vi "Cimb Set Modes.vi"   [LabVIEW 2016]
uses:
  Climb Control Type.ctl
  Climb Globals.vi
types:
  T1 = typedef "Climb Control Type.ctl" = enum16{"No Op", "Up", "Down"}
  T2 = typedef "Climb Notifier.ctl" = cluster{"Up":bool, "Down":bool, "Climb Control List":T1}
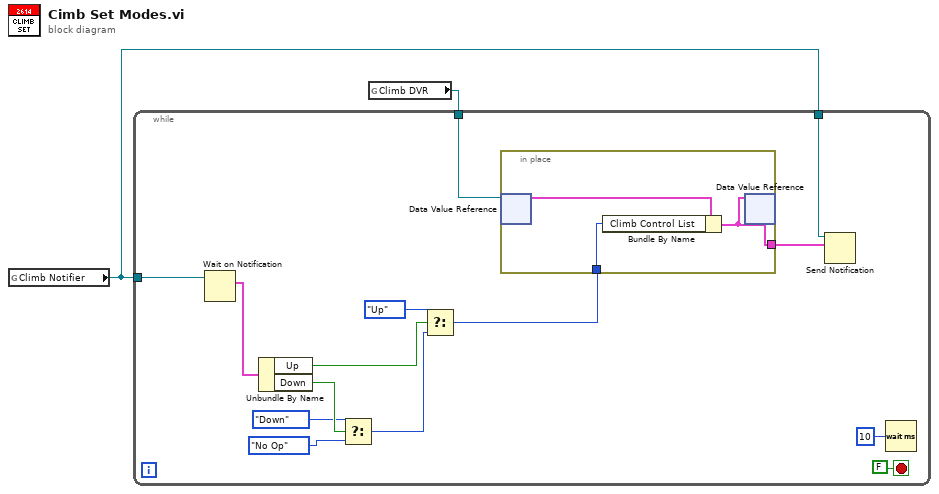
[diagram p0: block diagram]
diagram:
  n1 = global read "Climb Globals.vi" "Climb Notifier"() -> (w1:refnum<notifier>)
  n2 = global read "Climb Globals.vi" "Climb DVR"() -> (w2:refnum<data-value>)
  n3 = while {
    tunnel: w1 -> [w10]
    tunnel: w2 -> [w9]
    tunnel: w1 -> [w6]
    stop <- FALSE stop-if-true
    n4 = Wait on Notification(notifier=w10) -> (notification=w14:T2)  [unwired: 3 in, 3 out]
    n5 = Unbundle By Name(w14) -> ("Up"=w13:bool, "Down"=w12:bool)
    n6 = Select(t=Climb_Control_Type."Down" ("Climb Control List"), s=w12, f=Climb_Control_Type."No Op" ("Climb Control List")) -> (s? t:f=w11:T1)
    n7 = Select(t=Climb_Control_Type."Up" ("Climb Control List"), s=w13, f=w11) -> (s? t:f=w8:T1)
    n8 = in-place {
      in-place-border: w8 -> [w17]
      in-place-border: [w18] -> w7
      n9 = in-place-dvr #1(w9) -> (w19:T2)  [unwired: 1 out]
      n10 = Bundle By Name(cluster=w19, "Climb Control List"=w17) -> (w18:T2)
      n11 = in-place-dvr #1(w18) -> ()  [unwired: 2 out]
    }
    n12 = Send Notification(notification=w7, notifier=w6) -> ()  [unwired: 1 in, 2 out]
    n13 = Wait (ms)(milliseconds to wait=u32 10) -> ()  [unwired: 1 out]
  }
